vi "KDB Connect.vi"(4 "DBLocation":path, 5 "SqlMapper Type":refnum<class "SqlMapper.lvclass">, 6 "TableMapping":T1[](array[typedef])=[{"Table"="<Default>", "TableType"=enum."Memory"}], 8 "error in (no error)":errorcluster, 10 "Connection String":string) -> (0 "error out":errorcluster, 3 "SqlMapper out":refnum<class "SqlMapper.lvclass">)   [LabVIEW 2020, in "ORM_DBC_Kdb.lvlib" / "DBC.lvclass"]
uses:
  DBC.lvclass
  <vilib>/Viviota/shared/ORM.lvlibp/ORM/SqlMapper/SqlMapper.lvclass
  kdb_TableInfo_cluster.ctl
  kdb_TableType_enum.ctl
  DBC.lvclass/DBC.ctl
  C:/Program Files/National Instruments/LabVIEW 2024/vi.lib/Viviota/shared/ORM.lvlibp/ORM/DbConnection/DbConnection.lvclass
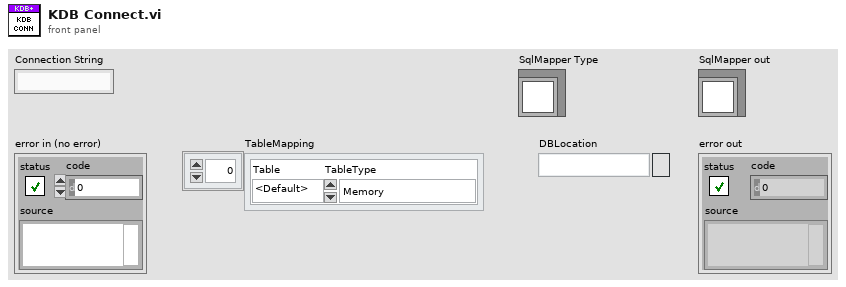
[diagram p1: front panel]
types:
  T1 = typedef "ORM_DBC_Kdb.lvlib/DBC.lvclass/kdb_TableInfo_cluster.ctl" = cluster{"Table":string, "TableType":T2}
  T2 = typedef "ORM_DBC_Kdb.lvlib/DBC.lvclass/kdb_TableType_enum.ctl" = enum16{"Memory", "Disk_Serialized", "Disk_Splayed", "Disk_Partitioned", "Other"}
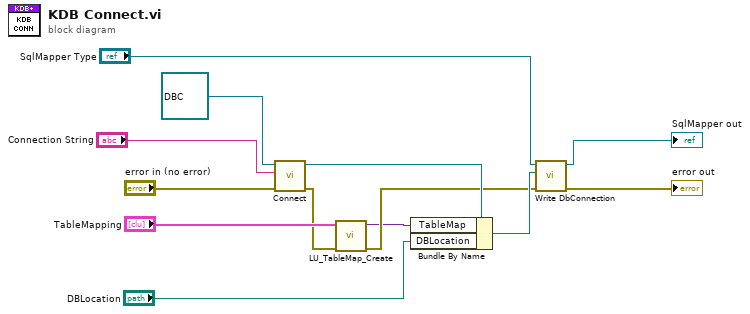
[diagram p0: block diagram]
diagram:
  n1 = call-dynamic "Connect.vi"("error in (no error)"="error in (no error)", "Connection String"="Connection String", "SqliteConnection in"=refnum<class "DBC.lvclass"> refnum ("KDBConnection.lvclass")) -> ("error out"=w6:errorcluster, "SqliteConnection out"=w5:refnum<class "DBC.lvclass">)  [unwired: 7 in]
  n2 = call "LU_TableMap_Create.vi"("error in"=w6, "TableMapping"="TableMapping") -> ("error out"=w3:errorcluster, "TableMap"=w2:variant)  [unwired: 8 in]
  n3 = Bundle By Name(cluster=w5, "TableMap"=w2, "DBLocation"="DBLocation") -> (w4:refnum<class "DBC.lvclass">)
  n4 = call <vilib>:"Write DbConnection.vi"("error in (no error)"=w3, "Dapper.lvlib:DbConnection.lvclass"=w4, "SqlMapper in"="SqlMapper Type") -> ("error out"=→"error out":errorcluster, "SqlMapper out"=→"SqlMapper out":refnum<class "SqlMapper.lvclass">)  [unwired: 7 in]
